vi "WaySensorTable (SubVI).vi"(10 "output cluster in":T1 {"UNDT_Cluster"."Gain Coeff" format="%#_6e"; "UNDT_Cluster"."Reserve 1" format="%02x"; "UNDT_Cluster"."Mux TX/RX" format="%02x"; "UNDT_Cluster"."ScanDelay" format="%02x"; "UNDT_Cluster"."PacketCounter" format="%08x"; "UNDT_Cluster"."SamplingInterval" format="%#_6e"; "UNDT_Cluster"."Lose Packet" format="%08x"; "UNDT_Cluster"."EncodersParam2" format="%016x"; "UNDT_Cluster"."EncodersParam1" format="%016x"; "UNDT_Cluster"."CRC 8" format="%02x"; "UNDT_Cluster"."N chanel" format="%02x"; "UNDT_Cluster"."N tick" format="%02x"; "UNDT_Cluster"."Ncycle" format="%04x"; "UNDT_Cluster"."FrameFormatVersion" format="%02x"; "UNDT_Cluster"."MagicWord" format="%.0x"}, 11 "MeasOut in":T3 {"FFT amplitude mean" format="%.2p"; "DC" format="%0.2p"; "time trig 2" format="%0.2p"; "time trig" format="%0.2p"; "detected frequency 2" format="%.2p"; "way sensor 2" format="%.2p"; "way sensor 1" format="%.2p"; "detected frequency" format="%.2p"; "RMS" format="%0.2p"; "amplitude" format="%.2p"; "FFT amplitude" format="%.2p"}) -> (3 "MeasOut out":T3 {"FFT amplitude mean" format="%.2p"; "DC" format="%0.2p"; "time trig 2" format="%0.2p"; "time trig" format="%0.2p"; "detected frequency 2" format="%.2p"; "way sensor 2" format="%.2p"; "way sensor 1" format="%.2p"; "detected frequency" format="%.2p"; "RMS" format="%0.2p"; "amplitude" format="%.2p"; "FFT amplitude" format="%.2p"})   [LabVIEW 2017]
uses:
  Control_EU/MeasControl.ctl
  Control_EU/DataCluster.ctl
  Control_EU/UNDT_ClusterPackRevers (Type).ctl
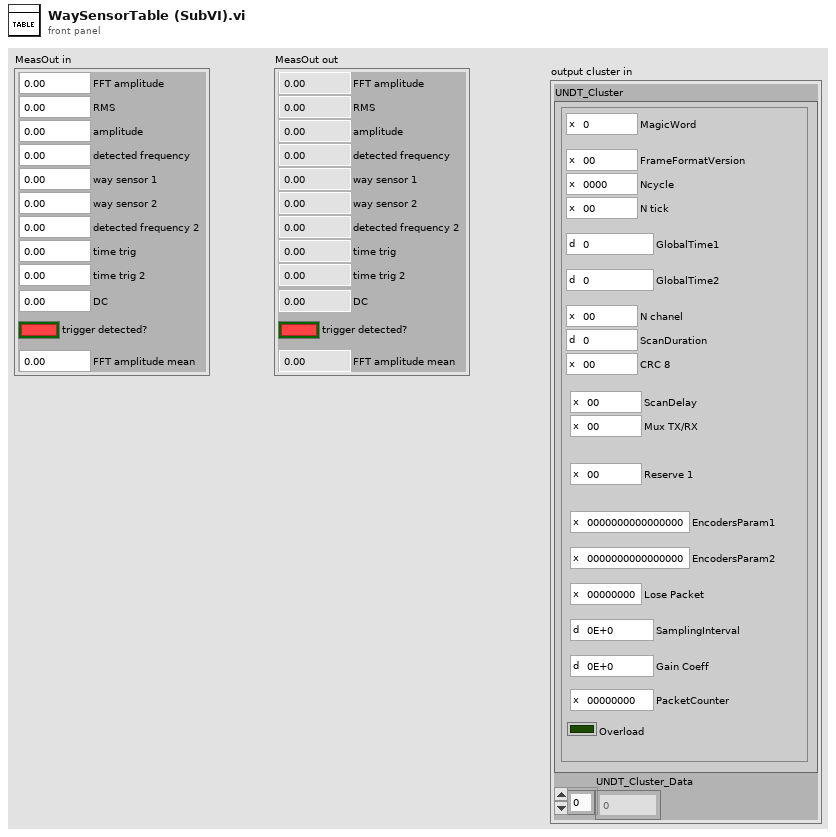
[diagram p1: front panel]
types:
  T1 = typedef "DataCluster.ctl" = cluster{"UNDT_Cluster":T2, "UNDT_Cluster_Data":dbl[]}
  T2 = typedef "UNDT_ClusterPackRevers (Type).ctl" = cluster{"PacketCounter":u32, "Gain Coeff":sgl, "SamplingInterval":sgl, "Lose Packet":u32, "EncodersParam2":u64, "EncodersParam1":u64, "Reserve 1":u8, "Mux TX/RX":u8, "ScanDelay":u16, "CRC 8":u8, "ScanDuration":u16, "N chanel":u8, "GlobalTime2":u32, "GlobalTime1":u32, "N tick":u8, "Ncycle":u16, "FrameFormatVersion":u8, "MagicWord":u32, "Overload":bool}
  T3 = typedef "MeasControl.ctl" = cluster{"FFT amplitude":dbl, "amplitude":dbl, "RMS":dbl, "detected frequency":dbl, "way sensor 1":ext, "way sensor 2":ext, "detected frequency 2":dbl, "time trig":dbl, "time trig 2":dbl, "DC":dbl, "trigger detected?":bool, "FFT amplitude mean":dbl}
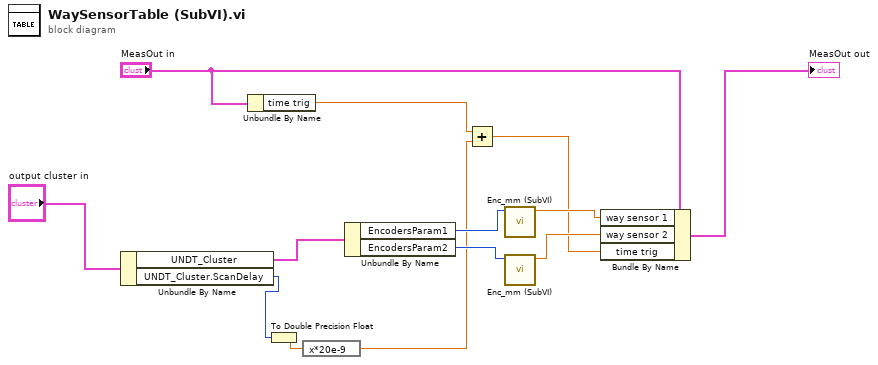
[diagram p0: block diagram]
diagram:
  n1 = Unbundle By Name("output cluster in") -> ("UNDT_Cluster"=w5:T2, "UNDT_Cluster.ScanDelay"=w7:u16)
  n2 = Unbundle By Name("MeasOut in") -> ("time trig"=w3:dbl)
  n3 = To Double Precision Float(number=w7) -> (double precision float=w8:dbl)
  n4 = expression code="x*20e-9"(w8) -> (w2:dbl)
  n5 = Unbundle By Name(w5) -> ("EncodersParam1"=w10:u64, "EncodersParam2"=w11:u64)
  n6 = Add(x=w3, y=w2) -> (x+y=w1:dbl)
  n7 = call "Enc_mm (SubVI).vi"("EncodersParam1"=w10) -> ("Numeric"=w13:ext)  [unwired: 10 in]
  n8 = call "Enc_mm (SubVI).vi"("EncodersParam1"=w11) -> ("Numeric"=w4:ext)  [unwired: 10 in]
  n9 = Bundle By Name(cluster="MeasOut in", "way sensor 1"=w13, "way sensor 2"=w4, "time trig"=w1) -> (→"MeasOut out":T3)
